vi "Read Test Display Raw.vi"(0 "VISA resource name":refnum<visa-resource-name>, 11 "error in (no error)":errorcluster) -> (4 "VISA resource name out":refnum<visa-resource-name>, 6 "Test Display Raw":string, 15 "error out":errorcluster)   [LabVIEW 2016, in "eec EST 300.lvlib"]
doc: "TD?\nReturns the raw unparsed string from the display. This can be used to monitor live readings during a test."
uses:
  <instrlib>/eec EST 300/eec EST 300.lvlib
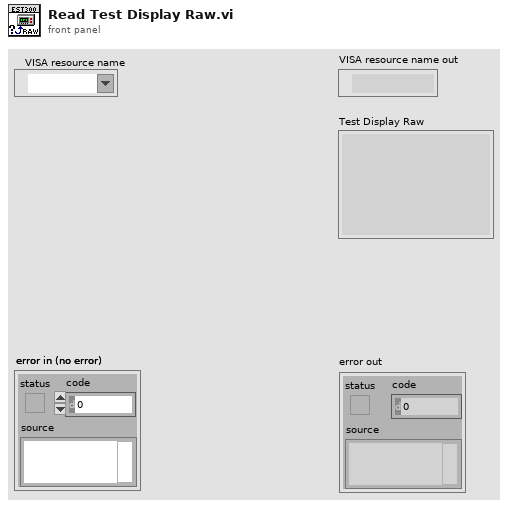
[diagram p1: front panel]
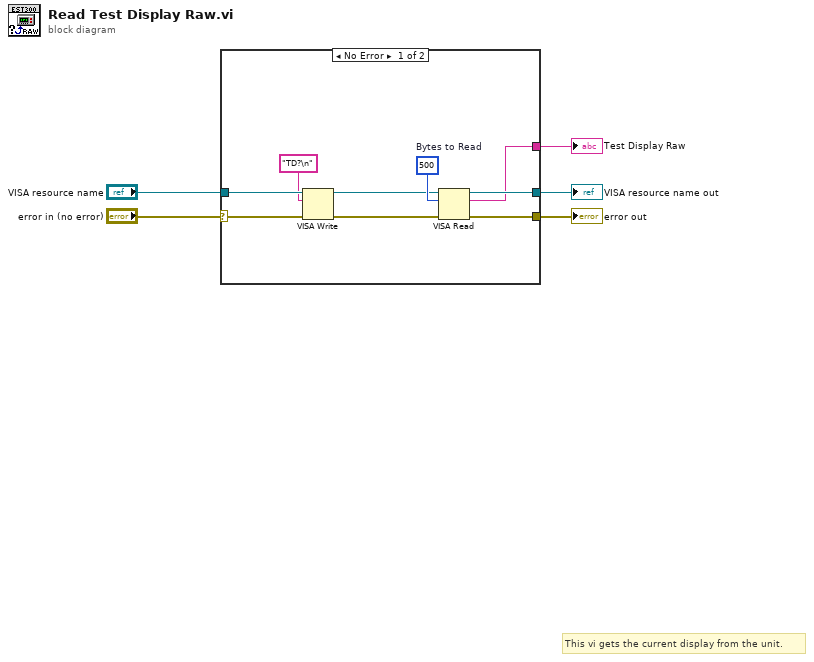
[diagram p0: block diagram]
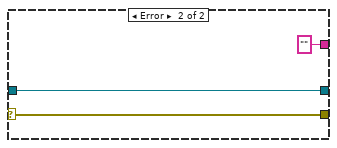
[diagram p2: hidden frame]
diagram:
  # "This vi gets the current display from the unit."
  n1 = case shown="No Error" "error in (no error)" {
    selector: "error in (no error)" -> [w14 w17]
    tunnel: [w10 w17] -> w4
    tunnel: [w7 w16] -> w2
    tunnel: "VISA resource name" -> [w13 w16]
    tunnel: [w6 "" ("read buffer")] -> w1
    frame No Error {
      w12 = u32 500  # Bytes to Read
      n2 = VISA Write(VISA resource name=w13, write buffer="TD?\n" ("string (\"\")"), error in (no error)=w14) -> (VISA resource name out=w9:refnum<visa-resource-name>, error out=w8:errorcluster)  [unwired: 1 out]
      n3 = VISA Read(VISA resource name=w9, byte count=w12, error in (no error)=w8) -> (VISA resource name out=w7:refnum<visa-resource-name>, read buffer=w6:string, error out=w10:errorcluster)  [unwired: 1 out]
    }
    frame Error {
    }
  }
  "error out" <- w4
  "VISA resource name out" <- w2
  "Test Display Raw" <- w1
